vi "GetCoEIndexOfTargetDevice.vi"() -> ()   [LabVIEW 2022 SP3]
panel:
  out "Device Address":string
  out "CoEIndexList":T1(array[cluster]) {"Object description"."Index" format="%x"}
  in  "EtherCAT Slave Address":string
  in  "CoE Index List":T2(ring)
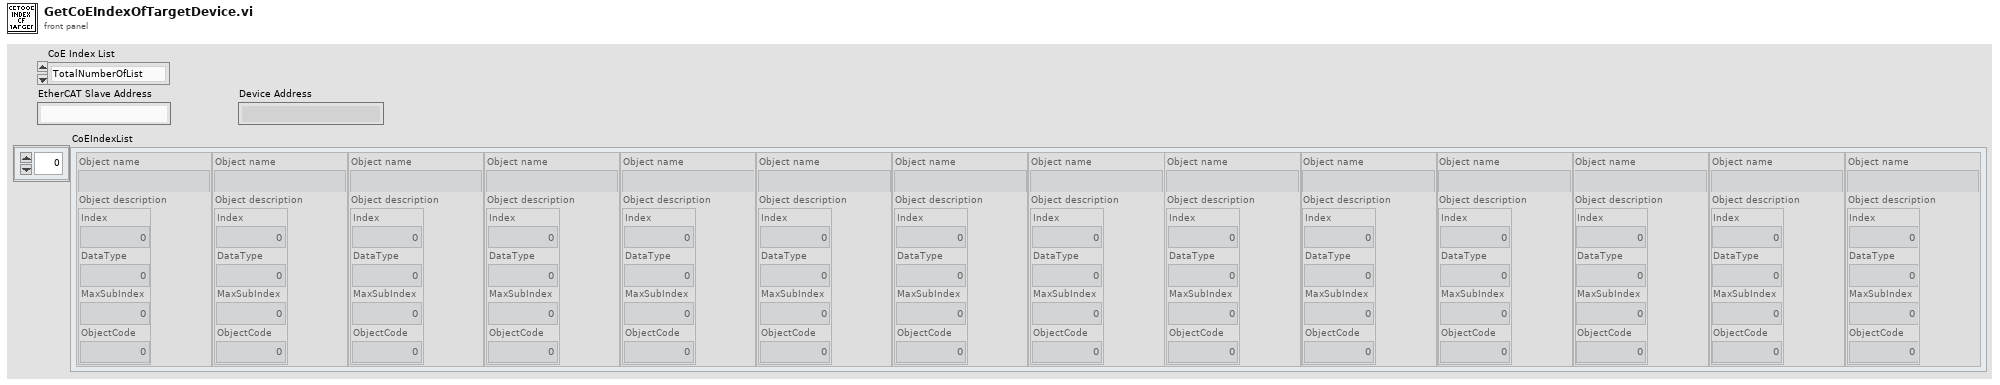
[diagram p1: front panel]
types:
  T1 = cluster{"Object name":string, "Object description":cluster{"Index":u16, "DataType":u16, "MaxSubIndex":u8, "ObjectCode":u16}}[]
  T2 = enum32{"TotalNumberOfList", "AllCoEObjects", "RxPDOs", "TxPDOs", "StoredForDevice", "StartUp"}
  T3 = cluster{"Index":u16, "DataType":u16, "MaxSubIndex":u8, "ObjectCode":u16}
  T4 = cluster{"Object name":string, "Object description":cluster{"Index":u16, "DataType":u16, "MaxSubIndex":u8, "ObjectCode":u16}}
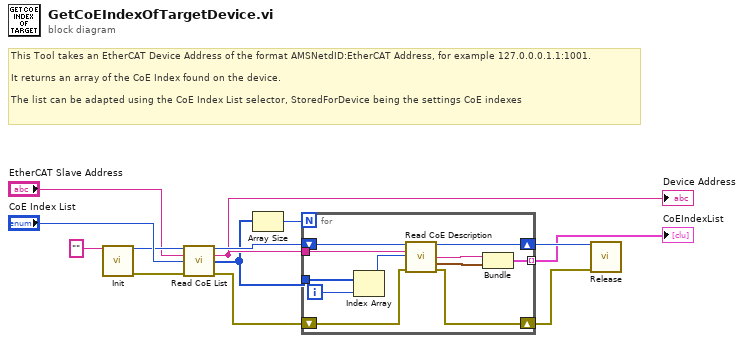
[diagram p0: block diagram]
diagram:
  # "This Tool takes an EtherCAT Device Address of the format AMSNetdID:EtherCAT Address, for example 127.0.0.0.1.1:1001.\n\nIt returns an array of the CoE Index found on the device.\n\nThe list can be adapted using the CoE Index List selector, StoredForDevice being the settings CoE indexes"
  n1 = call <userlib>:"Init.vi"("XMLDescription"="") -> ("Handle"=w12:u32, "error out"=w9:errorcluster)  [unwired: 10 in, 3 out]
  n2 = call <userlib>:"Read CoE List.vi"("Handle"=w12, "Device address"="EtherCAT Slave Address", "List type"="CoE Index List", "error in (no error)"=w9) -> ("Handle"=w8:u32, "Device address"=w6:string, "List"=w2:u16[], "error out"=w7:errorcluster)  [unwired: 8 in]
  "Device Address" <- w6
  n3 = Array Size(array=w2) -> (size(s)=w3:i32)
  n4 = for {
    N: w3 -> [_]
    tunnel: w6 -> [w22]
    shift-right: [w21] -> w5
    shift-left: w8 -> [w24]
    shift-right: [w20] -> w4
    shift-left: w7 -> [w23]
    tunnel: [w16] -> w1 mode=indexing
    tunnel: w2 -> [w19]
    i -> [w18]
    n5 = Index Array(array=w19, index=w18) -> (element=w17:u16)
    n6 = call <userlib>:"Read CoE Description.vi"("Handle"=w24, "Device address"=w22, "Index"=w17, "error in (no error)"=w23) -> ("Handle"=w21:u32, "Object name"=w15:string, "Object description"=w14:T3, "error out"=w20:errorcluster)  [unwired: 7 in, 1 out]
    n7 = Bundle("Object name"=w15, "Object description"=w14) -> (w16:T4)  [unwired: 1 in]
  }
  "CoEIndexList" <- w1
  n8 = call <userlib>:"Release.vi"("Handle"=w5, "error in (no error)"=w4) -> ()  [unwired: 13 in, 1 out]
